vi "P1Y3.vi"() -> ()   [LabVIEW 2020]
panel:
  out "Suhtarv":dbl
  in  "s":bool
  in  "autode arv 2":i32
  in  "leibkonna suurus1 2":dbl
  in  "lemmikloomad 2":i64
  in  "on õpilane1? 2":bool
  in  "perekonnanimi1 2":string
  in  "eesnimi1 2":string
  in  "autode arv":i32
  in  "leibkonna suurus1":dbl
  in  "lemmikloomad":i64
  in  "on õpilane1?":bool
  in  "perekonnanimi1":string
  in  "eesnimi1":string
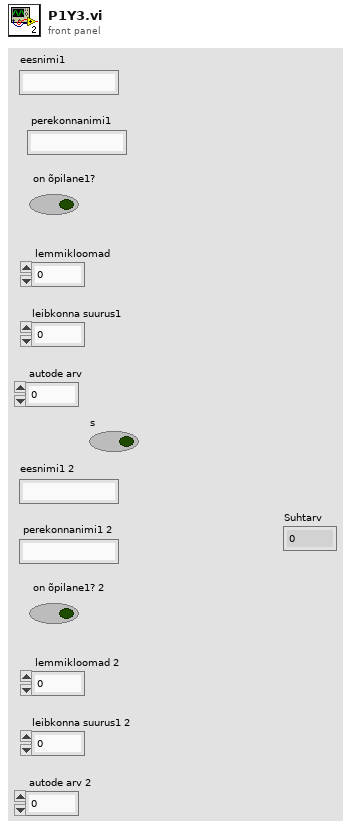
[diagram p1: front panel]
types:
  T1 = cluster{"eesnimi1":string, " perekonnanimi1":string, " on õpilane1?":bool, " lemmikloomad":i64, "leibkonna suurus1":dbl, " autode arv":i32}
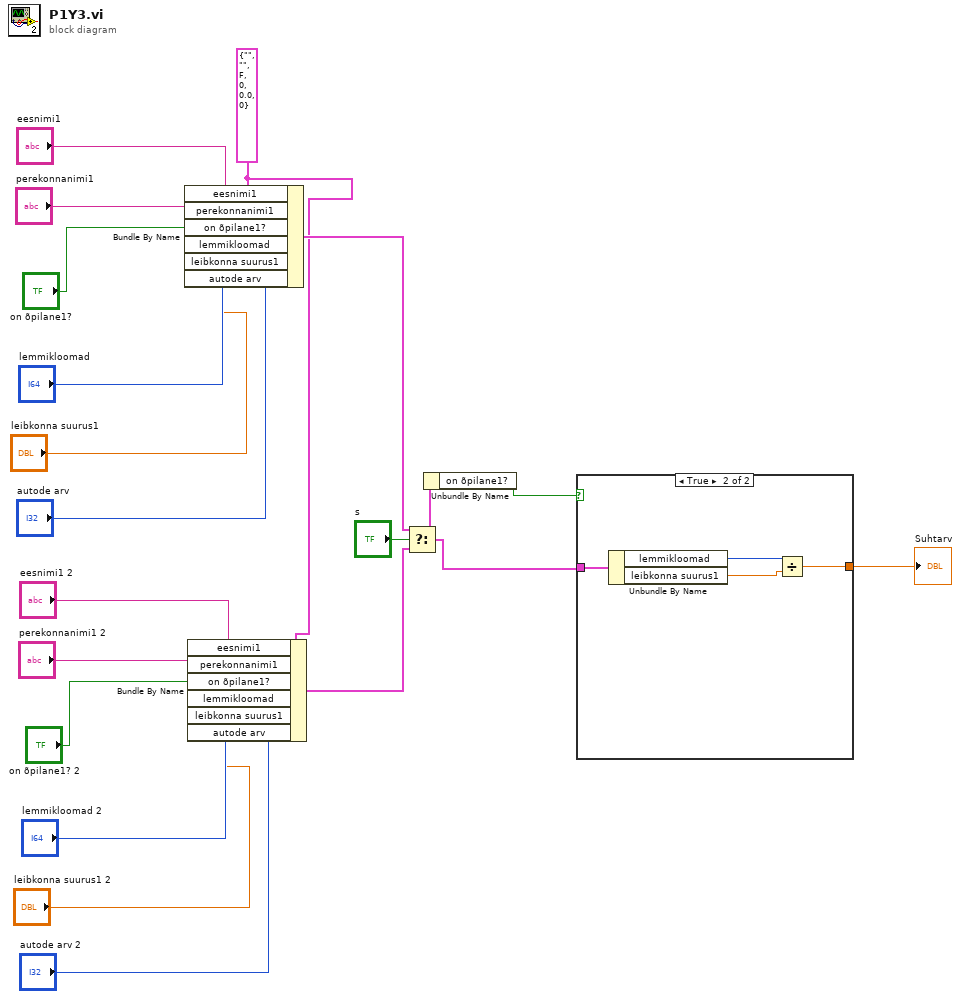
[diagram p0: block diagram]
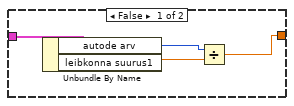
[diagram p2: hidden frame]
diagram:
  w1 = T1 {"eesnimi1"="", " perekonnanimi1"="", " on õpilane1?"=FALSE, " lemmikloomad"=0, "leibkonna suurus1"=0.0, " autode arv"=0} ("cluster")
  n1 = Bundle By Name(cluster=w1, "eesnimi1"="eesnimi1", "perekonnanimi1"="perekonnanimi1", "on õpilane1?"="on õpilane1?", "lemmikloomad"="lemmikloomad", "leibkonna suurus1"="leibkonna suurus1", "autode arv"="autode arv") -> (w6:T1)
  n2 = Bundle By Name(cluster=w1, "eesnimi1"="eesnimi1 2", "perekonnanimi1"="perekonnanimi1 2", "on õpilane1?"="on õpilane1? 2", "lemmikloomad"="lemmikloomad 2", "leibkonna suurus1"="leibkonna suurus1 2", "autode arv"="autode arv 2") -> (w5:T1)
  n3 = Select(t=w6, s="s", f=w5) -> (s? t:f=w3:T1)
  n4 = Unbundle By Name(w3) -> ("on õpilane1?"=w4:bool)
  n5 = case shown="True" w4 {
    tunnel: w3 -> [w23 w27]
    tunnel: [w20 w24] -> w2
    frame False {
      n6 = Unbundle By Name(w23) -> ("autode arv"=w22:i32, "leibkonna suurus1"=w21:dbl)
      n7 = Divide(x=w22, y=w21) -> (x/y=w20:dbl)
    }
    frame True {
      n8 = Unbundle By Name(w27) -> ("lemmikloomad"=w26:i64, "leibkonna suurus1"=w25:dbl)
      n9 = Divide(x=w26, y=w25) -> (x/y=w24:dbl)
    }
  }
  "Suhtarv" <- w2
